vi "update indices and next state.vi"(8 "error in":errorcluster, 11 "Simple Sequencer TBM runtime in":refnum<class "Simple Sequencer TBM runtime.lvclass">) -> (0 "error out":errorcluster, 3 "Simple Sequencer TBM runtime out":refnum<class "Simple Sequencer TBM runtime.lvclass">)   [LabVIEW 2014, in "Simple Sequencer TBM runtime.lvclass"]
doc: "This VI increments the Action pointer to point to the next Action in the Sequence. \nIf the Sequence is complete, it resets the Action pointer and points to the next Sequence in the Sequence list. \nIf it was the last Sequence in the list, then it either stops the sequences or starts over at the beginning depending on whether or not it was configured to repeat."
uses:
  Simple Sequencer TBM runtime.lvclass
  Simple Sequencer TBM runtime.lvclass/Simple Sequencer TBM runtime.ctl
  sequencer states.ctl
  sequencer commands.ctl
  <vilib>/NI/AMC/Create Single Message.vi
  <vilib>/NI/AMC/Update Message Routing Info.vi
  <vilib>/NI/AMC/Read Termination Message.vi
  <vilib>/NI/AMC/Send Message.vi
  <vilib>/NI/AMC/Globals.vi
  <vilib>/NI/AMC/AMC.lvlib
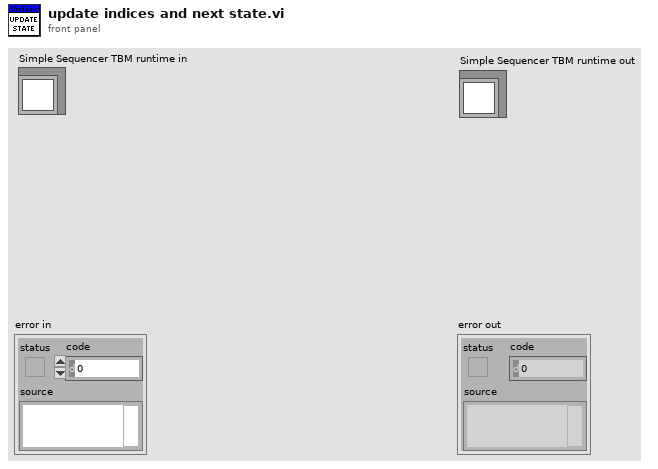
[diagram p1: front panel]
types:
  T1 = typedef "Simple Sequencer TBM runtime.lvclass/sequence definition.ctl" = cluster{"sequence name":string, "sequence length":i32, "actions with configuration":T2[]}
  T2 = typedef "Simple Sequencer TBM runtime.lvclass/actions with configuration.ctl" = cluster{"action":refnum<class "action.lvclass">, "parameters":T3, "parameters specification":T4[], "results":T3, "results specification":T4[]}
  T3 = typedef "tag bus.lvlib/data table.lvlib/data table.ctl" = cluster{"Double":dbl[], "Single":sgl[], "I64":i64[], "I32":i32[], "I16":i16[], "I8":i8[], "U64":u64[], "U32":u32[], "U16":u16[], "U8":u8[], "Boolean":bool[], "String":string[], "Array of Double":cluster{"DBL Array":dbl[]}[], "Array of Single":cluster{"SGL Array":sgl[]}[], "Array of I64":cluster{"I64 Array":i64[]}[], "Array of I32":cluster{"I32 Array":i32[]}[], "Array of I16":cluster{"I16 Array":i16[]}[], "Array of I8":cluster{"I8 Array":i8[]}[], "Array of U64":cluster{"U64 Array":u64[]}[], "Array of U32":cluster{"U32 Array":u32[]}[], "Array of U16":cluster{"U16 Array":u16[]}[], "Array of U8":cluster{"U8 Array":u8[]}[], "Array of Boolean":cluster{"Boolean Array":bool[]}[], "Array of String":cluster{"String Array":string[]}[]}
  T4 = typedef "tag bus.lvlib/data table.lvlib/transfer specification.ctl" = cluster{"data type":T5, "sink indices":i32[], "source indices":i32[]}
  T5 = typedef "tag bus.lvlib/tag descriptor.lvclass/Data Type.ctl" = enum16{"Double", "Single", "I64", "I32", "I16", "I8", "U64", "U32", "U16", "U8", "Boolean", "String", "Array of Double", "Array of Single", "Array of I64", "Array of I32", "Array of I16", "Array of I8", "Array of U64", "Array of U32", "Array of U16", "Array of U8", "Array of Boolean", "Array of String"}
  T6 = typedef "AMC.lvlib/Message Queue.ctl" = refnum<queue>
  T7 = typedef "Simple Sequencer TBM runtime.lvclass/sequencer states.ctl" = enum16{"stopped", "running", "paused"}
  T8 = typedef "Simple Sequencer TBM runtime.lvclass/sequencer commands.ctl" = enum16{"Run", "Pause", "Resume", "Stop"}
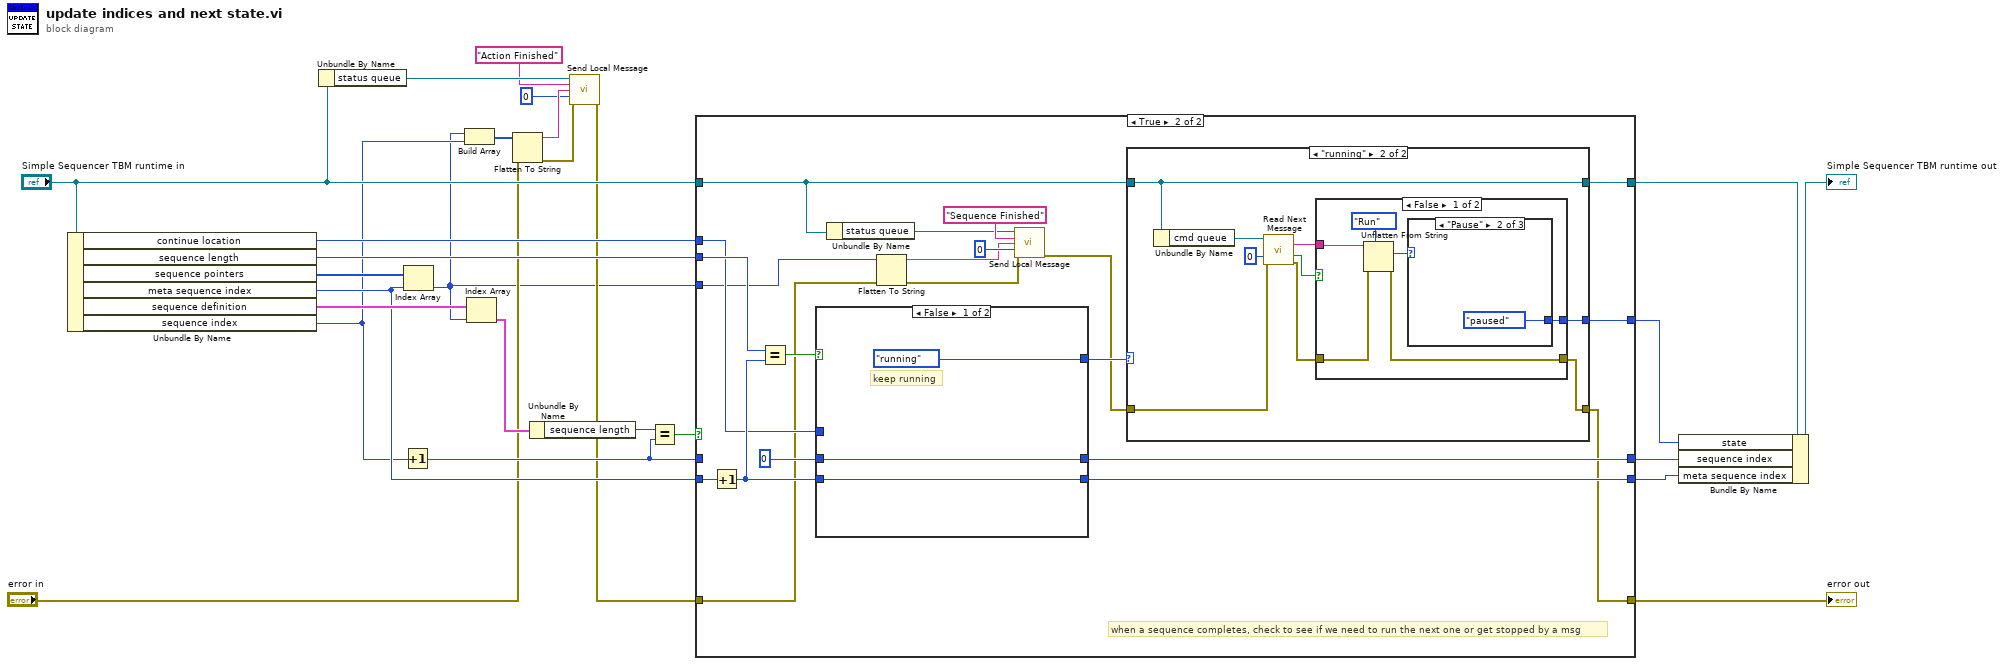
[diagram p0: block diagram]
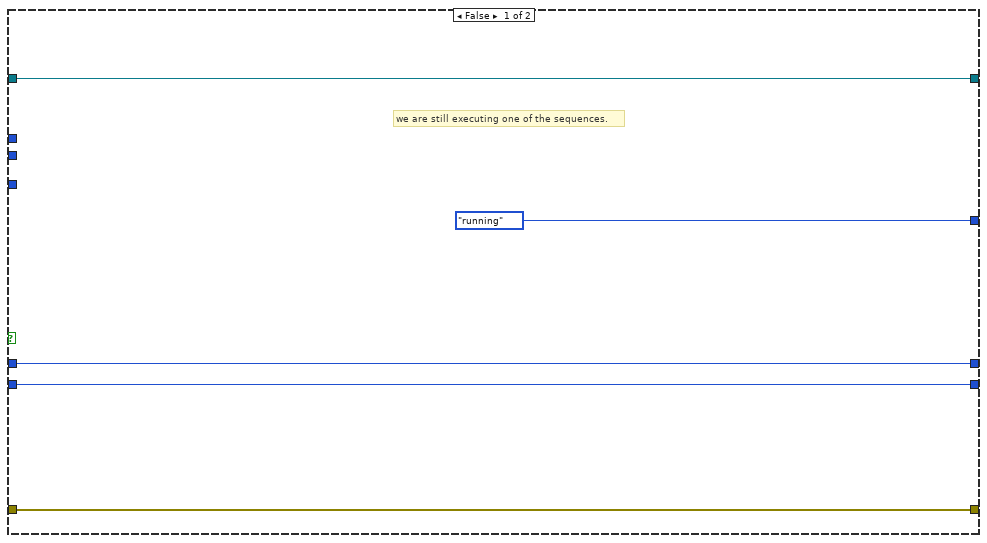
[diagram p2: hidden frame]
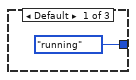
[diagram p4: hidden frame]
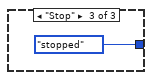
[diagram p5: hidden frame]
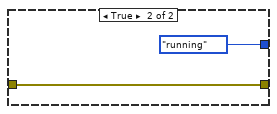
[diagram p6: hidden frame]
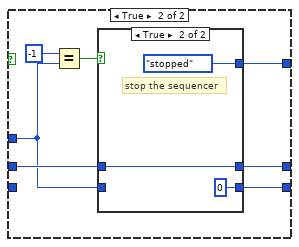
[diagram p7: hidden frame]
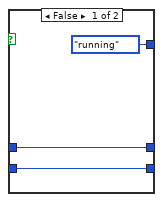
[diagram p8: hidden frame]
diagram:
  n1 = Unbundle By Name("Simple Sequencer TBM runtime in") -> ("continue location"=w19:i32, "sequence length"=w20:i32, "sequence pointers"=w26:i32[], "meta sequence index"=w7:i32, "sequence definition"=w25:T1[], "sequence index"=w6:i32)
  n2 = Unbundle By Name("Simple Sequencer TBM runtime in") -> ("status queue"=w10:T6)
  n3 = Increment(x=w6) -> (x+1=w21:i32)
  n4 = Index Array(array=w26, index=w7) -> (element=w1:i32)
  n5 = Build Array(w1, w6) -> (w14:i32[])
  n6 = Index Array(array=w25, index=w1) -> (element=w24:T1)
  n7 = Flatten To String(anything=w14, error in (no error)="error in") -> (data string=w12:string, error out=w13:errorcluster)  [unwired: 2 in, 1 out]
  n8 = Unbundle By Name(w24) -> ("sequence length"=w23:i32)
  n9 = call <vilib>:"Send Local Message.vi"("message queue in"=w10, "message name"="Action Finished", "message value"=w12, "timeout (-1 ms)"=0, "error in"=w13) -> ("error out"=w5:errorcluster)  [unwired: 8 in, 2 out]
  n10 = Equal?(x=w23, y=w21) -> (x = y?=w22:bool)
  n11 = case shown="True" w22 {
    tunnel: w21 -> [w31 _]
    tunnel: [w31 w46] -> w18
    tunnel: w7 -> [w30 w41]
    tunnel: [w30 w47] -> w17
    tunnel: w20 -> [_ w52]
    tunnel: w19 -> [_ w48]
    tunnel: [sequencer_states."running" w44] -> w16
    tunnel: "Simple Sequencer TBM runtime in" -> [w28 w35]
    tunnel: [w28 w43] -> w3
    tunnel: w5 -> [w27 w34]
    tunnel: [w27 w42] -> w2
    tunnel: w1 -> [_ w32]
    frame False {
      # "we are still executing one of the sequences."
    }
    frame True {
      # "when a sequence completes, check to see if we need to run the next one or get stopped by a msg"
      n12 = Increment(x=w41) -> (x+1=w50:i32)
      n13 = Equal?(x=w52, y=w50) -> (x = y?=w51:bool)
      n14 = case shown="False" w51 {
        tunnel: w50 -> [w77 _]
        tunnel: 0 -> [w78 w83]
        tunnel: w48 -> [_ w80]
        tunnel: [w77 w81] -> w47
        tunnel: [w78 w82] -> w46
        tunnel: [sequencer_states."running" w79] -> w45
        frame False {
          # "keep running"
        }
        frame True {
          n15 = Equal?(x=-1, y=w80) -> (x = y?=w84:bool)
          n16 = case shown="True" w84 {
            tunnel: w83 -> [w88 w91]
            tunnel: [w88 w91] -> w82
            tunnel: [w87 0 ("continue location")] -> w81
            tunnel: w80 -> [w87 _]
            tunnel: [sequencer_states."running" sequencer_states."stopped"] -> w79
            frame False {
            }
            frame True {
              # "stop the sequencer"
            }
          }
        }
      }
      n17 = Unbundle By Name(w35) -> ("status queue"=w36:T6)
      n18 = Flatten To String(anything=w32, error in (no error)=w34) -> (data string=w37:string, error out=w38:errorcluster)  [unwired: 2 in, 1 out]
      n19 = call <vilib>:"Send Local Message.vi"("message queue in"=w36, "message name"="Sequence Finished", "message value"=w37, "timeout (-1 ms)"=0, "error in"=w38) -> ("error out"=w33:errorcluster)  [unwired: 8 in, 2 out]
      n20 = case shown="\"running\"" w45 {
        selector: w45 -> [w55 _]
        tunnel: [w55 w59] -> w44
        tunnel: w35 -> [w54 w64]
        tunnel: [w54 w64] -> w43
        tunnel: w33 -> [w53 w62]
        tunnel: [w53 w56] -> w42
        frame "stopped", Default {
        }
        frame "running" {
          n21 = Unbundle By Name(w64) -> ("cmd queue"=w63:T6)
          n22 = call <vilib>:"Read Next Message.vi"("message queue in"=w63, "timeout (1 ms)"=0, "error in"=w62) -> ("message name"=w57:string, "timed out?"=w60:bool, "error out"=w58:errorcluster)  [unwired: 5 in, 5 out]
          n23 = case shown="False" w60 {
            tunnel: [w70 sequencer_states."running"] -> w59
            tunnel: w58 -> [w67 w74]
            tunnel: w57 -> [w68 _]
            tunnel: [w66 w74] -> w56
            frame False {
              n24 = Unflatten From String(type=sequencer_commands."Run" ("Commands"), binary string=w68, error in (no error)=w67) -> (value=w65:T8, error out=w66:errorcluster)  [unwired: 2 in, 1 out]
              n25 = case shown="\"Pause\"" w65 {
                tunnel: [sequencer_states."running" sequencer_states."paused" sequencer_states."stopped"] -> w70
                frame Default {
                }
                frame "Pause" {
                }
                frame "Stop" {
                }
              }
            }
            frame True {
            }
          }
        }
      }
    }
  }
  "error out" <- w2
  n26 = Bundle By Name(cluster=w3, "state"=w16, "sequence index"=w18, "meta sequence index"=w17) -> (→"Simple Sequencer TBM runtime out":refnum<class "Simple Sequencer TBM runtime.lvclass">)
